vi "layout.vi"(0 "reference":refnum<class "InitialStateNode.lvclass">, 1 "graph":refnum<class "Graph.lvclass">, 2 "graphics":refnum<class "Graphics.lvclass">, 3 "grid":refnum<class "Grid.lvclass">, 5 "error in (no error)":errorcluster) -> (14 "reference out":refnum<class "InitialStateNode.lvclass">, 19 "error out":errorcluster)   [LabVIEW 2020, in "InitialStateNode.lvclass"]
doc: "public void layout(Graph g, Graphics2D g2, Grid grid)"
uses:
  <resource>/Framework/Providers/Open_GDS/UML/InitialStateNode_class/InitialStateNode.lvclass
  C:/Program Files (x86)/National Instruments/LabVIEW 2020/resource/Framework/Providers/Open_GDS/UML/RectangularNode_class/RectangularNode.lvclass
  <resource>/Framework/Providers/Open_GDS/UML/Graph_class/Graph.lvclass
  <resource>/Framework/Providers/Open_GDS/UML/Graphics_class/Graphics.lvclass
  <resource>/Framework/Providers/Open_GDS/UML/Grid_class/Grid.lvclass
  <resource>/Framework/Providers/Open_GDS/UML/RectangularNode_class/RectangularNode.lvclass
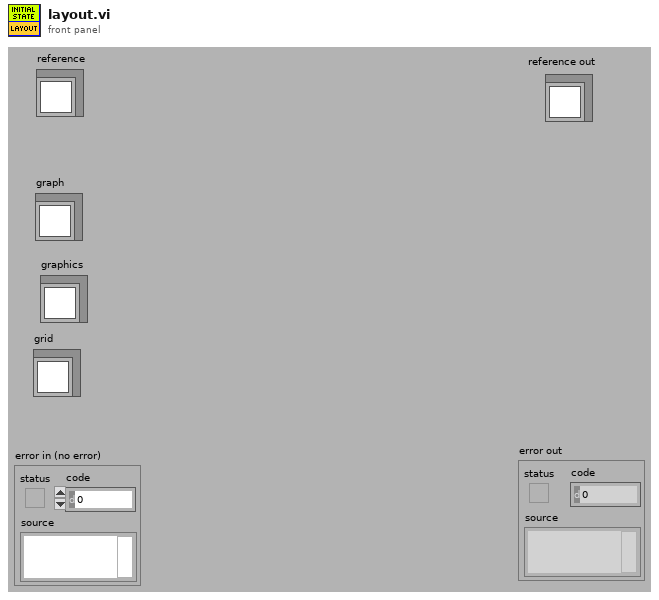
[diagram p1: front panel]
types:
  T1 = typedef "RectangularNode.lvclass/ObjectAttributes.ctl" = cluster{"bounds":T2}
  T2 = typedef "Rectangle Rectangle2D.ctl" = cluster{"x":dbl, "y":dbl, "width":dbl, "height":dbl}
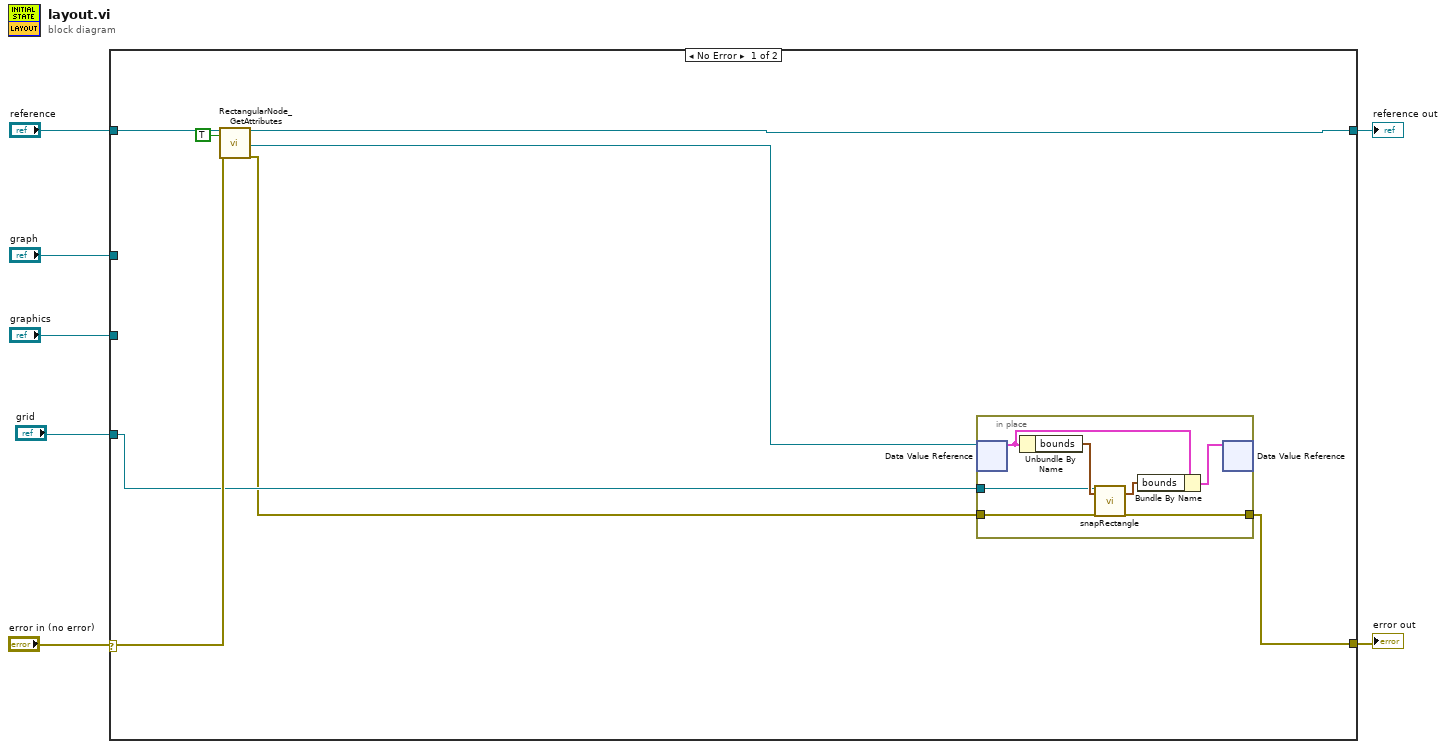
[diagram p0: block diagram]
diagram:
  n1 = case shown="No Error" "error in (no error)" {
    selector: "error in (no error)" -> [w13 w23]
    tunnel: "reference" -> [w15 w24]
    tunnel: [w8 w23] -> w6
    tunnel: [w14 w24] -> w5
    tunnel: "graph" -> [_ _]
    tunnel: "graphics" -> [_ _]
    tunnel: "grid" -> [w10 _]
    frame No Error {
      n2 = call <resource>:"RectangularNode_GetAttributes.vi"("reference in"=w15, "OnlyGetDvrReference(False)"=TRUE, "error in (no error)"=w13) -> ("reference out"=w14:refnum<class "InitialStateNode.lvclass">, "DataRef"=w11:refnum<data-value>, "error out"=w9:errorcluster)  [unwired: 13 in, 1 out]
      n3 = in-place {
        in-place-border: w10 -> [w18]
        in-place-border: w9 -> [w17]
        in-place-border: [w16] -> w8
        n4 = in-place-dvr #1(w11) -> (w22:T1)  [unwired: 1 out]
        n5 = Unbundle By Name(w22) -> ("bounds"=w19:T2)
        n6 = call <resource>:"snapRectangle.vi"("reference"=w18, "bounds"=w19, "error in (no error)"=w17) -> ("boundsOut"=w21:T2, "error out"=w16:errorcluster)  [unwired: 15 out]
        n7 = Bundle By Name(cluster=w22, "bounds"=w21) -> (w20:T1)
        n8 = in-place-dvr #1(w20) -> ()  [unwired: 2 out]
      }
    }
    frame Error {
    }
  }
  "reference out" <- w5
  "error out" <- w6
